vi "Test - Draw Teapot.vi"() -> ()   [LabVIEW 2022 SP3, in "Raster.lvlib"]
uses:
  Raster.lvlib
  3D/Triangle.ctl
  3D/Vertex.ctl
  3D/Vector 3D.ctl
  UV.ctl
  Rectangle Dimensions.ctl
  5ea285c7-be76-47ab-bb95-511c6a9aac96.vi
  d84cddbd-8e40-43c7-a758-6e8d8fd6f2c6.vi
  <vilib>/Utility/High Resolution Relative Seconds.vi
  Sort Points.vi
  Calc P4.vi
  Draw Flat Bottom Filled Triangle.vi
  Draw Flat Top Filled Triangle.vi
  Draw Horizontal Line.vi
  3D/Round Vertex.vi
  Utility/Convert Pixels To Picture.vi/d601d993-a776-4dc8-89c7-357d8398c88c.vi
  Utility/Convert Pixels To Picture.vi/7816d0d6-8e4d-41a2-85ac-ed82f1435763.vi
  Round SGL.vi
  Draw Flat Bottom Filled Triangle.vi/c0c82237-b583-4fc1-b44f-40d02a28ecfd.vi
  Draw Flat Bottom Filled Triangle.vi/53435b12-820c-4aea-aec4-7de16a894549.vi
  Calc Triangle Line Reciprocals.vi
  Global 1.vi
  <vilib>/Utility/colorconv.llb/Color to RGB.vi
  <vilib>/Utility/colorconv.llb/RGB to Color.vi
  <vilib>/picture/picture.llb/Draw Unflattened Pixmap.vi
  <vilib>/picture/picture.llb/Draw True-Color Pixmap.vi
  Utility/Utility.lvlib
  3D/3D.lvlib
panel:
  out "Pixel count":u32
  in  "Teapot":T1[](array[typedef])=[{"Vertex 1"={"Position"={"x"=400.0, "y"=370.36023, "z"=0.9922247}, "UV"={"u"=0.0, "v"=0.0}, "Colour"=12517256}, "Vertex 2"={"Position"={"x"=400.0, "y"=370.5378, "z"=0.99224055}, "UV"={"u"=0.0, "v"=0.0}, "Colour"=12517256}, "Vertex 3"={"Position"={"x"=418.7357, "y"=370.73743, "z"=0.99221843}, "UV"={"u"=0.0, "v"=0.0}, "Colour"=12517256}, "Alpha"=0.0, "Alpha Blending Enabled"=FALSE, "Colour"=11067768}, {"Vertex 1"={"Position"={"x"=400.0, "y"=365.60147, "z"=0.9922195}, "UV"={"u"=0.0, "v"=0.0}, "Colour"=12517256}, "Vertex 2"={"Position"={"x"=400.0, "y"=362.58005, "z"=0.99223673}, "UV"={"u"=0.0, "v"=0.0}, "Colour"=12517256}, "Vertex 3"={"Position"={"x"=381.29703, "y"=362.75687, "z"=0.9922147}, "UV"={"u"=0.0, "v"=0.0}, "Colour"=12517256}, "Alpha"=0.0, "Alpha Blending Enabled"=FALSE, "Colour"=4941110}, {"Vertex 1"={"Position"={"x"=400.0, "y"=370.5378, "z"=0.99224055}, "UV"={"u"=0.0, "v"=0.0}, "Colour"=12517256}, "Vertex 2"={"Position"={"x"=400.0, "y"=370.36023, "z"=0.9922247}, "UV"={"u"=0.0, "v"=0.0}, "Colour"=12517256}, "Vertex 3"={"Position"={"x"=381.39975, "y"=370.55798, "z"=0.99220276}, "UV"={"u"=0.0, "v"=0.0}, "Colour"=12517256}, "Alpha"=0.0, "Alpha Blending Enabled"=FALSE, "Colour"=11067768}, {"Vertex 1"={"Position"={"x"=381.39975, "y"=370.55798, "z"=0.99220276}, "UV"={"u"=0.0, "v"=0.0}, "Colour"=12517256}, "Vertex 2"={"Position"={"x"=381.2643, "y"=370.73743, "z"=0.99221843}, "UV"={"u"=0.0, "v"=0.0}, "Colour"=12517256}, "Vertex 3"={"Position"={"x"=400.0, "y"=370.5378, "z"=0.99224055}, "UV"={"u"=0.0, "v"=0.0}, "Colour"=12517256}, "Alpha"=0.0, "Alpha Blending Enabled"=FALSE, "Colour"=11067768}, {"Vertex 1"={"Position"={"x"=400.0, "y"=362.58005, "z"=0.99223673}, "UV"={"u"=0.0, "v"=0.0}, "Colour"=12517256}, "Vertex 2"={"Position"={"x"=400.0, "y"=365.60147, "z"=0.9922195}, "UV"={"u"=0.0, "v"=0.0}, "Colour"=12517256}, "Vertex 3"={"Position"={"x"=418.5554, "y"=365.78537, "z"=0.9921976}, "UV"={"u"=0.0, "v"=0.0}, "Colour"=12517256}, "Alpha"=0.0, "Alpha Blending Enabled"=FALSE, "Colour"=4941110}, {"Vertex 1"={"Position"={"x"=418.5554, "y"=365.78537, "z"=0.9921976}, "UV"={"u"=0.0, "v"=0.0}, "Colour"=12517256}, "Vertex 2"={"Position"={"x"=418.70297, "y"=362.75687, "z"=0.9922147}, "UV"={"u"=0.0, "v"=0.0}, "Colour"=12517256}, "Vertex 3"={"Position"={"x"=400.0, "y"=362.58005, "z"=0.99223673}, "UV"={"u"=0.0, "v"=0.0}, "Colour"=12517256}, "Alpha"=0.0, "Alpha Blending Enabled"=FALSE, "Colour"=4941110}, {"Vertex 1"={"Position"={"x"=418.7357, "y"=370.73743, "z"=0.99221843}, "UV"={"u"=0.0, "v"=0.0}, "Colour"=12517256}, "Vertex 2"={"Position"={"x"=418.60028, "y"=370.55798, "z"=0.99220276}, "UV"={"u"=0.0, "v"=0.0}, "Colour"=12517256}, "Vertex 3"={"Position"={"x"=400.0, "y"=370.36023, "z"=0.9922247}, "UV"={"u"=0.0, "v"=0.0}, "Colour"=12517256}, "Alpha"=0.0, "Alpha Blending Enabled"=FALSE, "Colour"=11067768}, {"Vertex 1"={"Position"={"x"=400.0, "y"=369.48642, "z"=0.992215}, "UV"={"u"=0.0, "v"=0.0}, "Colour"=12517256}, "Vertex 2"={"Position"={"x"=400.0, "y"=370.36023, "z"=0.9922247}, "UV"={"u"=0.0, "v"=0.0}, "Colour"=12517256}, "Vertex 3"={"Position"={"x"=418.60028, "y"=370.55798, "z"=0.99220276}, "UV"={"u"=0.0, "v"=0.0}, "Colour"=12517256}, "Alpha"=0.0, "Alpha Blending Enabled"=FALSE, "Colour"=12253829}, {"Vertex 1"={"Position"={"x"=400.0, "y"=370.36023, "z"=0.9922247}, "UV"={"u"=0.0, "v"=0.0}, "Colour"=12517256}, "Vertex 2"={"Position"={"x"=400.0, "y"=369.48642, "z"=0.992215}, "UV"={"u"=0.0, "v"=0.0}, "Colour"=12517256}, "Vertex 3"={"Position"={"x"=381.4836, "y"=369.6808, "z"=0.9921931}, "UV"={"u"=0.0, "v"=0.0}, "Colour"=12517256}, "Alpha"=0.0, "Alpha Blending Enabled"=FALSE, "Colour"=12253829}, {"Vertex 1"={"Position"={"x"=381.29703, "y"=362.75687, "z"=0.9922147}, "UV"={"u"=0.0, "v"=0.0}, "Colour"=12517256}, "Vertex 2"={"Position"={"x"=381.4446, "y"=365.78537, "z"=0.9921976}, "UV"={"u"=0.0, "v"=0.0}, "Colour"=12517256}, "Vertex 3"={"Position"={"x"=400.0, "y"=365.60147, "z"=0.9922195}, "UV"={"u"=0.0, "v"=0.0}, "Colour"=12517256}, "Alpha"=0.0, "Alpha Blending Enabled"=FALSE, "Colour"=4941110}, {"Vertex 1"={"Position"={"x"=400.0, "y"=367.90298, "z"=0.9922127}, "UV"={"u"=0.0, "v"=0.0}, "Colour"=12517256}, "Vertex 2"={"Position"={"x"=400.0, "y"=365.60147, "z"=0.9922195}, "UV"={"u"=0.0, "v"=0.0}, "Colour"=12517256}, "Vertex 3"={"Position"={"x"=381.4446, "y"=365.78537, "z"=0.9921976}, "UV"={"u"=0.0, "v"=0.0}, "Colour"=12517256}, "Alpha"=0.0, "Alpha Blending Enabled"=FALSE, "Colour"=6917451}, {"Vertex 1"={"Position"={"x"=400.0, "y"=365.60147, "z"=0.9922195}, "UV"={"u"=0.0, "v"=0.0}, "Colour"=12517256}, "Vertex 2"={"Position"={"x"=400.0, "y"=367.90298, "z"=0.9922127}, "UV"={"u"=0.0, "v"=0.0}, "Colour"=12517256}, "Vertex 3"={"Position"={"x"=418.49722, "y"=368.09274, "z"=0.99219084}, "UV"={"u"=0.0, "v"=0.0}, "Colour"=12517256}, "Alpha"=0.0, "Alpha Blending Enabled"=FALSE, "Colour"=6917451}, {"Vertex 1"={"Position"={"x"=400.0, "y"=367.90298, "z"=0.9922127}, "UV"={"u"=0.0, "v"=0.0}, "Colour"=12517256}, "Vertex 2"={"Position"={"x"=400.0, "y"=369.48642, "z"=0.992215}, "UV"={"u"=0.0, "v"=0.0}, "Colour"=12517256}, "Vertex 3"={"Position"={"x"=418.5164, "y"=369.6808, "z"=0.9921931}, "UV"={"u"=0.0, "v"=0.0}, "Colour"=12517256}, "Alpha"=0.0, "Alpha Blending Enabled"=FALSE, "Colour"=9618536}, {"Vertex 1"={"Position"={"x"=381.4836, "y"=369.6808, "z"=0.9921931}, "UV"={"u"=0.0, "v"=0.0}, "Colour"=12517256}, "Vertex 2"={"Position"={"x"=381.39975, "y"=370.55798, "z"=0.99220276}, "UV"={"u"=0.0, "v"=0.0}, "Colour"=12517256}, "Vertex 3"={"Position"={"x"=400.0, "y"=370.36023, "z"=0.9922247}, "UV"={"u"=0.0, "v"=0.0}, "Colour"=12517256}, "Alpha"=0.0, "Alpha Blending Enabled"=FALSE, "Colour"=12253829}, {"Vertex 1"={"Position"={"x"=400.0, "y"=369.48642, "z"=0.992215}, "UV"={"u"=0.0, "v"=0.0}, "Colour"=12517256}, "Vertex 2"={"Position"={"x"=400.0, "y"=367.90298, "z"=0.9922127}, "UV"={"u"=0.0, "v"=0.0}, "Colour"=12517256}, "Vertex 3"={"Position"={"x"=381.50278, "y"=368.09274, "z"=0.99219084}, "UV"={"u"=0.0, "v"=0.0}, "Colour"=12517256}, "Alpha"=0.0, "Alpha Blending Enabled"=FALSE, "Colour"=9618536}, {"Vertex 1"={"Position"={"x"=418.60028, "y"=370.55798, "z"=0.99220276}, "UV"={"u"=0.0, "v"=0.0}, "Colour"=12517256}, "Vertex 2"={"Position"={"x"=418.5164, "y"=369.6808, "z"=0.9921931}, "UV"={"u"=0.0, "v"=0.0}, "Colour"=12517256}, "Vertex 3"={"Position"={"x"=400.0, "y"=369.48642, "z"=0.992215}, "UV"={"u"=0.0, "v"=0.0}, "Colour"=12517256}, "Alpha"=0.0, "Alpha Blending Enabled"=FALSE, "Colour"=12253829}, {"Vertex 1"={"Position"={"x"=418.49722, "y"=368.09274, "z"=0.99219084}, "UV"={"u"=0.0, "v"=0.0}, "Colour"=12517256}, "Vertex 2"={"Position"={"x"=418.5554, "y"=365.78537, "z"=0.9921976}, "UV"={"u"=0.0, "v"=0.0}, "Colour"=12517256}, "Vertex 3"={"Position"={"x"=400.0, "y"=365.60147, "z"=0.9922195}, "UV"={"u"=0.0, "v"=0.0}, "Colour"=12517256}, "Alpha"=0.0, "Alpha Blending Enabled"=FALSE, "Colour"=6917451}, {"Vertex 1"={"Position"={"x"=381.4446, "y"=365.78537, "z"=0.9921976}, "UV"={"u"=0.0, "v"=0.0}, "Colour"=12517256}, "Vertex 2"={"Position"={"x"=381.50278, "y"=368.09274, "z"=0.99219084}, "UV"={"u"=0.0, "v"=0.0}, "Colour"=12517256}, "Vertex 3"={"Position"={"x"=400.0, "y"=367.90298, "z"=0.9922127}, "UV"={"u"=0.0, "v"=0.0}, "Colour"=12517256}, "Alpha"=0.0, "Alpha Blending Enabled"=FALSE, "Colour"=6917451}, {"Vertex 1"={"Position"={"x"=381.50278, "y"=368.09274, "z"=0.99219084}, "UV"={"u"=0.0, "v"=0.0}, "Colour"=12517256}, "Vertex 2"={"Position"={"x"=381.4836, "y"=369.6808, "z"=0.9921931}, "UV"={"u"=0.0, "v"=0.0}, "Colour"=12517256}, "Vertex 3"={"Position"={"x"=400.0, "y"=369.48642, "z"=0.992215}, "UV"={"u"=0.0, "v"=0.0}, "Colour"=12517256}, "Alpha"=0.0, "Alpha Blending Enabled"=FALSE, "Colour"=9618536}, {"Vertex 1"={"Position"={"x"=418.5164, "y"=369.6808, "z"=0.9921931}, "UV"={"u"=0.0, "v"=0.0}, "Colour"=12517256}, "Vertex 2"={"Position"={"x"=418.49722, "y"=368.09274, "z"=0.99219084}, "UV"={"u"=0.0, "v"=0.0}, "Colour"=12517256}, "Vertex 3"={"Position"={"x"=400.0, "y"=367.90298, "z"=0.9922127}, "UV"={"u"=0.0, "v"=0.0}, "Colour"=12517256}, "Alpha"=0.0, "Alpha Blending Enabled"=FALSE, "Colour"=9618536}, {"Vertex 1"={"Position"={"x"=418.60028, "y"=370.55798, "z"=0.99220276}, "UV"={"u"=0.0, "v"=0.0}, "Colour"=12517256}, "Vertex 2"={"Position"={"x"=418.7357, "y"=370.73743, "z"=0.99221843}, "UV"={"u"=0.0, "v"=0.0}, "Colour"=12517256}, "Vertex 3"={"Position"={"x"=436.73154, "y"=371.323, "z"=0.99215364}, "UV"={"u"=0.0, "v"=0.0}, "Colour"=12517256}, "Alpha"=0.0, "Alpha Blending Enabled"=FALSE, "Colour"=11001975}, {"Vertex 1"={"Position"={"x"=381.4446, "y"=365.78537, "z"=0.9921976}, "UV"={"u"=0.0, "v"=0.0}, "Colour"=12517256}, "Vertex 2"={"Position"={"x"=381.29703, "y"=362.75687, "z"=0.9922147}, "UV"={"u"=0.0, "v"=0.0}, "Colour"=12517256}, "Vertex 3"={"Position"={"x"=363.33307, "y"=363.27545, "z"=0.99214995}, "UV"={"u"=0.0, "v"=0.0}, "Colour"=12517256}, "Alpha"=0.0, "Alpha Blending Enabled"=FALSE, "Colour"=4743475}, {"Vertex 1"={"Position"={"x"=381.2643, "y"=370.73743, "z"=0.99221843}, "UV"={"u"=0.0, "v"=0.0}, "Colour"=12517256}, "Vertex 2"={"Position"={"x"=381.39975, "y"=370.55798, "z"=0.99220276}, "UV"={"u"=0.0, "v"=0.0}, "Colour"=12517256}, "Vertex 3"={"Position"={"x"=363.53616, "y"=371.13776, "z"=0.99213827}, "UV"={"u"=0.0, "v"=0.0}, "Colour"=12517256}, "Alpha"=0.0, "Alpha Blending Enabled"=FALSE, "Colour"=11001975}, {"Vertex 1"={"Position"={"x"=418.70297, "y"=362.75687, "z"=0.9922147}, "UV"={"u"=0.0, "v"=0.0}, "Colour"=12517256}, "Vertex 2"={"Position"={"x"=418.5554, "y"=365.78537, "z"=0.9921976}, "UV"={"u"=0.0, "v"=0.0}, "Colour"=12517256}, "Vertex 3"={"Position"={"x"=436.37515, "y"=366.32462, "z"=0.9921332}, "UV"={"u"=0.0, "v"=0.0}, "Colour"=12517256}, "Alpha"=0.0, "Alpha Blending Enabled"=FALSE, "Colour"=4743475}, {"Vertex 1"={"Position"={"x"=418.5164, "y"=369.6808, "z"=0.9921931}, "UV"={"u"=0.0, "v"=0.0}, "Colour"=12517256}, "Vertex 2"={"Position"={"x"=418.60028, "y"=370.55798, "z"=0.99220276}, "UV"={"u"=0.0, "v"=0.0}, "Colour"=12517256}, "Vertex 3"={"Position"={"x"=436.46384, "y"=371.13776, "z"=0.99213827}, "UV"={"u"=0.0, "v"=0.0}, "Colour"=12517256}, "Alpha"=0.0, "Alpha Blending Enabled"=FALSE, "Colour"=12056195}, {"Vertex 1"={"Position"={"x"=381.39975, "y"=370.55798, "z"=0.99220276}, "UV"={"u"=0.0, "v"=0.0}, "Colour"=12517256}, "Vertex 2"={"Position"={"x"=381.4836, "y"=369.6808, "z"=0.9921931}, "UV"={"u"=0.0, "v"=0.0}, "Colour"=12517256}, "Vertex 3"={"Position"={"x"=363.7018, "y"=370.25076, "z"=0.9921288}, "UV"={"u"=0.0, "v"=0.0}, "Colour"=12517256}, "Alpha"=0.0, "Alpha Blending Enabled"=FALSE, "Colour"=12056195}, {"Vertex 1"={"Position"={"x"=381.50278, "y"=368.09274, "z"=0.99219084}, "UV"={"u"=0.0, "v"=0.0}, "Colour"=12517256}, "Vertex 2"={"Position"={"x"=381.4446, "y"=365.78537, "z"=0.9921976}, "UV"={"u"=0.0, "v"=0.0}, "Colour"=12517256}, "Vertex 3"={"Position"={"x"=363.62485, "y"=366.32462, "z"=0.9921332}, "UV"={"u"=0.0, "v"=0.0}, "Colour"=12517256}, "Alpha"=0.0, "Alpha Blending Enabled"=FALSE, "Colour"=6719817}, {"Vertex 1"={"Position"={"x"=418.5554, "y"=365.78537, "z"=0.9921976}, "UV"={"u"=0.0, "v"=0.0}, "Colour"=12517256}, "Vertex 2"={"Position"={"x"=418.49722, "y"=368.09274, "z"=0.99219084}, "UV"={"u"=0.0, "v"=0.0}, "Colour"=12517256}, "Vertex 3"={"Position"={"x"=436.26022, "y"=368.64917, "z"=0.9921266}, "UV"={"u"=0.0, "v"=0.0}, "Colour"=12517256}, "Alpha"=0.0, "Alpha Blending Enabled"=FALSE, "Colour"=6719817}, {"Vertex 1"={"Position"={"x"=418.49722, "y"=368.09274, "z"=0.99219084}, "UV"={"u"=0.0, "v"=0.0}, "Colour"=12517256}, "Vertex 2"={"Position"={"x"=418.5164, "y"=369.6808, "z"=0.9921931}, "UV"={"u"=0.0, "v"=0.0}, "Colour"=12517256}, "Vertex 3"={"Position"={"x"=436.2982, "y"=370.25076, "z"=0.9921288}, "UV"={"u"=0.0, "v"=0.0}, "Colour"=12517256}, "Alpha"=0.0, "Alpha Blending Enabled"=FALSE, "Colour"=9355110}, {"Vertex 1"={"Position"={"x"=381.4836, "y"=369.6808, "z"=0.9921931}, "UV"={"u"=0.0, "v"=0.0}, "Colour"=12517256}, "Vertex 2"={"Position"={"x"=381.50278, "y"=368.09274, "z"=0.99219084}, "UV"={"u"=0.0, "v"=0.0}, "Colour"=12517256}, "Vertex 3"={"Position"={"x"=363.73975, "y"=368.64917, "z"=0.9921266}, "UV"={"u"=0.0, "v"=0.0}, "Colour"=12517256}, "Alpha"=0.0, "Alpha Blending Enabled"=FALSE, "Colour"=9355110}, {"Vertex 1"={"Position"={"x"=363.53616, "y"=371.13776, "z"=0.99213827}, "UV"={"u"=0.0, "v"=0.0}, "Colour"=12517256}, "Vertex 2"={"Position"={"x"=363.26846, "y"=371.323, "z"=0.99215364}, "UV"={"u"=0.0, "v"=0.0}, "Colour"=12517256}, "Vertex 3"={"Position"={"x"=381.2643, "y"=370.73743, "z"=0.99221843}, "UV"={"u"=0.0, "v"=0.0}, "Colour"=12517256}, "Alpha"=0.0, "Alpha Blending Enabled"=FALSE, "Colour"=11001975}, {"Vertex 1"={"Position"={"x"=436.37515, "y"=366.32462, "z"=0.9921332}, "UV"={"u"=0.0, "v"=0.0}, "Colour"=12517256}, "Vertex 2"={"Position"={"x"=436.66693, "y"=363.27545, "z"=0.99214995}, "UV"={"u"=0.0, "v"=0.0}, "Colour"=12517256}, "Vertex 3"={"Position"={"x"=418.70297, "y"=362.75687, "z"=0.9922147}, "UV"={"u"=0.0, "v"=0.0}, "Colour"=12517256}, "Alpha"=0.0, "Alpha Blending Enabled"=FALSE, "Colour"=4743475}, {"Vertex 1"={"Position"={"x"=436.73154, "y"=371.323, "z"=0.99215364}, "UV"={"u"=0.0, "v"=0.0}, "Colour"=12517256}, "Vertex 2"={"Position"={"x"=436.46384, "y"=371.13776, "z"=0.99213827}, "UV"={"u"=0.0, "v"=0.0}, "Colour"=12517256}, "Vertex 3"={"Position"={"x"=418.60028, "y"=370.55798, "z"=0.99220276}, "UV"={"u"=0.0, "v"=0.0}, "Colour"=12517256}, "Alpha"=0.0, "Alpha Blending Enabled"=FALSE, "Colour"=11001975}, {"Vertex 1"={"Position"={"x"=363.33307, "y"=363.27545, "z"=0.99214995}, "UV"={"u"=0.0, "v"=0.0}, "Colour"=12517256}, "Vertex 2"={"Position"={"x"=363.62485, "y"=366.32462, "z"=0.9921332}, "UV"={"u"=0.0, "v"=0.0}, "Colour"=12517256}, "Vertex 3"={"Position"={"x"=381.4446, "y"=365.78537, "z"=0.9921976}, "UV"={"u"=0.0, "v"=0.0}, "Colour"=12517256}, "Alpha"=0.0, "Alpha Blending Enabled"=FALSE, "Colour"=4743475}, {"Vertex 1"={"Position"={"x"=363.7018, "y"=370.25076, "z"=0.9921288}, "UV"={"u"=0.0, "v"=0.0}, "Colour"=12517256}, "Vertex 2"={"Position"={"x"=363.53616, "y"=371.13776, "z"=0.99213827}, "UV"={"u"=0.0, "v"=0.0}, "Colour"=12517256}, "Vertex 3"={"Position"={"x"=381.39975, "y"=370.55798, "z"=0.99220276}, "UV"={"u"=0.0, "v"=0.0}, "Colour"=12517256}, "Alpha"=0.0, "Alpha Blending Enabled"=FALSE, "Colour"=12056195}, {"Vertex 1"={"Position"={"x"=436.46384, "y"=371.13776, "z"=0.99213827}, "UV"={"u"=0.0, "v"=0.0}, "Colour"=12517256}, "Vertex 2"={"Position"={"x"=436.2982, "y"=370.25076, "z"=0.9921288}, "UV"={"u"=0.0, "v"=0.0}, "Colour"=12517256}, "Vertex 3"={"Position"={"x"=418.5164, "y"=369.6808, "z"=0.9921931}, "UV"={"u"=0.0, "v"=0.0}, "Colour"=12517256}, "Alpha"=0.0, "Alpha Blending Enabled"=FALSE, "Colour"=12056195}, {"Vertex 1"={"Position"={"x"=436.26022, "y"=368.64917, "z"=0.9921266}, "UV"={"u"=0.0, "v"=0.0}, "Colour"=12517256}, "Vertex 2"={"Position"={"x"=436.37515, "y"=366.32462, "z"=0.9921332}, "UV"={"u"=0.0, "v"=0.0}, "Colour"=12517256}, "Vertex 3"={"Position"={"x"=418.5554, "y"=365.78537, "z"=0.9921976}, "UV"={"u"=0.0, "v"=0.0}, "Colour"=12517256}, "Alpha"=0.0, "Alpha Blending Enabled"=FALSE, "Colour"=6719817}, {"Vertex 1"={"Position"={"x"=363.62485, "y"=366.32462, "z"=0.9921332}, "UV"={"u"=0.0, "v"=0.0}, "Colour"=12517256}, "Vertex 2"={"Position"={"x"=363.73975, "y"=368.64917, "z"=0.9921266}, "UV"={"u"=0.0, "v"=0.0}, "Colour"=12517256}, "Vertex 3"={"Position"={"x"=381.50278, "y"=368.09274, "z"=0.99219084}, "UV"={"u"=0.0, "v"=0.0}, "Colour"=12517256}, "Alpha"=0.0, "Alpha Blending Enabled"=FALSE, "Colour"=6719817}, {"Vertex 1"={"Position"={"x"=363.73975, "y"=368.64917, "z"=0.9921266}, "UV"={"u"=0.0, "v"=0.0}, "Colour"=12517256}, "Vertex 2"={"Position"={"x"=363.7018, "y"=370.25076, "z"=0.9921288}, "UV"={"u"=0.0, "v"=0.0}, "Colour"=12517256}, "Vertex 3"={"Position"={"x"=381.4836, "y"=369.6808, "z"=0.9921931}, "UV"={"u"=0.0, "v"=0.0}, "Colour"=12517256}, "Alpha"=0.0, "Alpha Blending Enabled"=FALSE, "Colour"=9355110}, {"Vertex 1"={"Position"={"x"=436.2982, "y"=370.25076, "z"=0.9921288}, "UV"={"u"=0.0, "v"=0.0}, "Colour"=12517256}, "Vertex 2"={"Position"={"x"=436.26022, "y"=368.64917, "z"=0.9921266}, "UV"={"u"=0.0, "v"=0.0}, "Colour"=12517256}, "Vertex 3"={"Position"={"x"=418.49722, "y"=368.09274, "z"=0.99219084}, "UV"={"u"=0.0, "v"=0.0}, "Colour"=12517256}, "Alpha"=0.0, "Alpha Blending Enabled"=FALSE, "Colour"=9355110}, {"Vertex 1"={"Position"={"x"=436.46384, "y"=371.13776, "z"=0.99213827}, "UV"={"u"=0.0, "v"=0.0}, "Colour"=12517256}, "Vertex 2"={"Position"={"x"=436.73154, "y"=371.323, "z"=0.99215364}, "UV"={"u"=0.0, "v"=0.0}, "Colour"=12517256}, "Vertex 3"={"Position"={"x"=454.01846, "y"=372.28268, "z"=0.99204737}, "UV"={"u"=0.0, "v"=0.0}, "Colour"=12517256}, "Alpha"=0.0, "Alpha Blending Enabled"=FALSE, "Colour"=10870134}, {"Vertex 1"={"Position"={"x"=363.62485, "y"=366.32462, "z"=0.9921332}, "UV"={"u"=0.0, "v"=0.0}, "Colour"=12517256}, "Vertex 2"={"Position"={"x"=363.33307, "y"=363.27545, "z"=0.99214995}, "UV"={"u"=0.0, "v"=0.0}, "Colour"=12517256}, "Vertex 3"={"Position"={"x"=346.07788, "y"=364.12534, "z"=0.9920438}, "UV"={"u"=0.0, "v"=0.0}, "Colour"=12517256}, "Alpha"=0.0, "Alpha Blending Enabled"=FALSE, "Colour"=4347951}, {"Vertex 1"={"Position"={"x"=363.26846, "y"=371.323, "z"=0.99215364}, "UV"={"u"=0.0, "v"=0.0}, "Colour"=12517256}, "Vertex 2"={"Position"={"x"=363.53616, "y"=371.13776, "z"=0.99213827}, "UV"={"u"=0.0, "v"=0.0}, "Colour"=12517256}, "Vertex 3"={"Position"={"x"=346.38046, "y"=372.08786, "z"=0.9920326}, "UV"={"u"=0.0, "v"=0.0}, "Colour"=12517256}, "Alpha"=0.0, "Alpha Blending Enabled"=FALSE, "Colour"=10870134}, {"Vertex 1"={"Position"={"x"=436.66693, "y"=363.27545, "z"=0.99214995}, "UV"={"u"=0.0, "v"=0.0}, "Colour"=12517256}, "Vertex 2"={"Position"={"x"=436.37515, "y"=366.32462, "z"=0.9921332}, "UV"={"u"=0.0, "v"=0.0}, "Colour"=12517256}, "Vertex 3"={"Position"={"x"=453.4873, "y"=367.20825, "z"=0.9920277}, "UV"={"u"=0.0, "v"=0.0}, "Colour"=12517256}, "Alpha"=0.0, "Alpha Blending Enabled"=FALSE, "Colour"=4347951}, {"Vertex 1"={"Position"={"x"=436.2982, "y"=370.25076, "z"=0.9921288}, "UV"={"u"=0.0, "v"=0.0}, "Colour"=12517256}, "Vertex 2"={"Position"={"x"=436.46384, "y"=371.13776, "z"=0.99213827}, "UV"={"u"=0.0, "v"=0.0}, "Colour"=12517256}, "Vertex 3"={"Position"={"x"=453.61954, "y"=372.08786, "z"=0.9920326}, "UV"={"u"=0.0, "v"=0.0}, "Colour"=12517256}, "Alpha"=0.0, "Alpha Blending Enabled"=FALSE, "Colour"=11726719}, {"Vertex 1"={"Position"={"x"=363.53616, "y"=371.13776, "z"=0.99213827}, "UV"={"u"=0.0, "v"=0.0}, "Colour"=12517256}, "Vertex 2"={"Position"={"x"=363.7018, "y"=370.25076, "z"=0.9921288}, "UV"={"u"=0.0, "v"=0.0}, "Colour"=12517256}, "Vertex 3"={"Position"={"x"=346.62732, "y"=371.18472, "z"=0.99202347}, "UV"={"u"=0.0, "v"=0.0}, "Colour"=12517256}, "Alpha"=0.0, "Alpha Blending Enabled"=FALSE, "Colour"=11726719}, {"Vertex 1"={"Position"={"x"=363.73975, "y"=368.64917, "z"=0.9921266}, "UV"={"u"=0.0, "v"=0.0}, "Colour"=12517256}, "Vertex 2"={"Position"={"x"=363.62485, "y"=366.32462, "z"=0.9921332}, "UV"={"u"=0.0, "v"=0.0}, "Colour"=12517256}, "Vertex 3"={"Position"={"x"=346.5127, "y"=367.20825, "z"=0.9920277}, "UV"={"u"=0.0, "v"=0.0}, "Colour"=12517256}, "Alpha"=0.0, "Alpha Blending Enabled"=FALSE, "Colour"=6258756}, {"Vertex 1"={"Position"={"x"=436.37515, "y"=366.32462, "z"=0.9921332}, "UV"={"u"=0.0, "v"=0.0}, "Colour"=12517256}, "Vertex 2"={"Position"={"x"=436.26022, "y"=368.64917, "z"=0.9921266}, "UV"={"u"=0.0, "v"=0.0}, "Colour"=12517256}, "Vertex 3"={"Position"={"x"=453.3161, "y"=369.56085, "z"=0.9920214}, "UV"={"u"=0.0, "v"=0.0}, "Colour"=12517256}, "Alpha"=0.0, "Alpha Blending Enabled"=FALSE, "Colour"=6258756}, {"Vertex 1"={"Position"={"x"=436.26022, "y"=368.64917, "z"=0.9921266}, "UV"={"u"=0.0, "v"=0.0}, "Colour"=12517256}, "Vertex 2"={"Position"={"x"=436.2982, "y"=370.25076, "z"=0.9921288}, "UV"={"u"=0.0, "v"=0.0}, "Colour"=12517256}, "Vertex 3"={"Position"={"x"=453.37268, "y"=371.18472, "z"=0.99202347}, "UV"={"u"=0.0, "v"=0.0}, "Colour"=12517256}, "Alpha"=0.0, "Alpha Blending Enabled"=FALSE, "Colour"=8959585}, {"Vertex 1"={"Position"={"x"=363.7018, "y"=370.25076, "z"=0.9921288}, "UV"={"u"=0.0, "v"=0.0}, "Colour"=12517256}, "Vertex 2"={"Position"={"x"=363.73975, "y"=368.64917, "z"=0.9921266}, "UV"={"u"=0.0, "v"=0.0}, "Colour"=12517256}, "Vertex 3"={"Position"={"x"=346.6839, "y"=369.56085, "z"=0.9920214}, "UV"={"u"=0.0, "v"=0.0}, "Colour"=12517256}, "Alpha"=0.0, "Alpha Blending Enabled"=FALSE, "Colour"=8959585}, {"Vertex 1"={"Position"={"x"=346.38046, "y"=372.08786, "z"=0.9920326}, "UV"={"u"=0.0, "v"=0.0}, "Colour"=12517256}, "Vertex 2"={"Position"={"x"=345.98154, "y"=372.28268, "z"=0.99204737}, "UV"={"u"=0.0, "v"=0.0}, "Colour"=12517256}, "Vertex 3"={"Position"={"x"=363.26846, "y"=371.323, "z"=0.99215364}, "UV"={"u"=0.0, "v"=0.0}, "Colour"=12517256}, "Alpha"=0.0, "Alpha Blending Enabled"=FALSE, "Colour"=10870134}, {"Vertex 1"={"Position"={"x"=453.4873, "y"=367.20825, "z"=0.9920277}, "UV"={"u"=0.0, "v"=0.0}, "Colour"=12517256}, "Vertex 2"={"Position"={"x"=453.92212, "y"=364.12534, "z"=0.9920438}, "UV"={"u"=0.0, "v"=0.0}, "Colour"=12517256}, "Vertex 3"={"Position"={"x"=436.66693, "y"=363.27545, "z"=0.99214995}, "UV"={"u"=0.0, "v"=0.0}, "Colour"=12517256}, "Alpha"=0.0, "Alpha Blending Enabled"=FALSE, "Colour"=4347951}, {"Vertex 1"={"Position"={"x"=454.01846, "y"=372.28268, "z"=0.99204737}, "UV"={"u"=0.0, "v"=0.0}, "Colour"=12517256}, "Vertex 2"={"Position"={"x"=453.61954, "y"=372.08786, "z"=0.9920326}, "UV"={"u"=0.0, "v"=0.0}, "Colour"=12517256}, "Vertex 3"={"Position"={"x"=436.46384, "y"=371.13776, "z"=0.99213827}, "UV"={"u"=0.0, "v"=0.0}, "Colour"=12517256}, "Alpha"=0.0, "Alpha Blending Enabled"=FALSE, "Colour"=10870134}, {"Vertex 1"={"Position"={"x"=346.07788, "y"=364.12534, "z"=0.9920438}, "UV"={"u"=0.0, "v"=0.0}, "Colour"=12517256}, "Vertex 2"={"Position"={"x"=346.5127, "y"=367.20825, "z"=0.9920277}, "UV"={"u"=0.0, "v"=0.0}, "Colour"=12517256}, "Vertex 3"={"Position"={"x"=363.62485, "y"=366.32462, "z"=0.9921332}, "UV"={"u"=0.0, "v"=0.0}, "Colour"=12517256}, "Alpha"=0.0, "Alpha Blending Enabled"=FALSE, "Colour"=4347951}, {"Vertex 1"={"Position"={"x"=346.62732, "y"=371.18472, "z"=0.99202347}, "UV"={"u"=0.0, "v"=0.0}, "Colour"=12517256}, "Vertex 2"={"Position"={"x"=346.38046, "y"=372.08786, "z"=0.9920326}, "UV"={"u"=0.0, "v"=0.0}, "Colour"=12517256}, "Vertex 3"={"Position"={"x"=363.53616, "y"=371.13776, "z"=0.99213827}, "UV"={"u"=0.0, "v"=0.0}, "Colour"=12517256}, "Alpha"=0.0, "Alpha Blending Enabled"=FALSE, "Colour"=11726719}, {"Vertex 1"={"Position"={"x"=453.61954, "y"=372.08786, "z"=0.9920326}, "UV"={"u"=0.0, "v"=0.0}, "Colour"=12517256}, "Vertex 2"={"Position"={"x"=453.37268, "y"=371.18472, "z"=0.99202347}, "UV"={"u"=0.0, "v"=0.0}, "Colour"=12517256}, "Vertex 3"={"Position"={"x"=436.2982, "y"=370.25076, "z"=0.9921288}, "UV"={"u"=0.0, "v"=0.0}, "Colour"=12517256}, "Alpha"=0.0, "Alpha Blending Enabled"=FALSE, "Colour"=11726719}, {"Vertex 1"={"Position"={"x"=453.3161, "y"=369.56085, "z"=0.9920214}, "UV"={"u"=0.0, "v"=0.0}, "Colour"=12517256}, "Vertex 2"={"Position"={"x"=453.4873, "y"=367.20825, "z"=0.9920277}, "UV"={"u"=0.0, "v"=0.0}, "Colour"=12517256}, "Vertex 3"={"Position"={"x"=436.37515, "y"=366.32462, "z"=0.9921332}, "UV"={"u"=0.0, "v"=0.0}, "Colour"=12517256}, "Alpha"=0.0, "Alpha Blending Enabled"=FALSE, "Colour"=6258756}, {"Vertex 1"={"Position"={"x"=346.5127, "y"=367.20825, "z"=0.9920277}, "UV"={"u"=0.0, "v"=0.0}, "Colour"=12517256}, "Vertex 2"={"Position"={"x"=346.6839, "y"=369.56085, "z"=0.9920214}, "UV"={"u"=0.0, "v"=0.0}, "Colour"=12517256}, "Vertex 3"={"Position"={"x"=363.73975, "y"=368.64917, "z"=0.9921266}, "UV"={"u"=0.0, "v"=0.0}, "Colour"=12517256}, "Alpha"=0.0, "Alpha Blending Enabled"=FALSE, "Colour"=6258756}, {"Vertex 1"={"Position"={"x"=346.6839, "y"=369.56085, "z"=0.9920214}, "UV"={"u"=0.0, "v"=0.0}, "Colour"=12517256}, "Vertex 2"={"Position"={"x"=346.62732, "y"=371.18472, "z"=0.99202347}, "UV"={"u"=0.0, "v"=0.0}, "Colour"=12517256}, "Vertex 3"={"Position"={"x"=363.7018, "y"=370.25076, "z"=0.9921288}, "UV"={"u"=0.0, "v"=0.0}, "Colour"=12517256}, "Alpha"=0.0, "Alpha Blending Enabled"=FALSE, "Colour"=8959585}, {"Vertex 1"={"Position"={"x"=453.37268, "y"=371.18472, "z"=0.99202347}, "UV"={"u"=0.0, "v"=0.0}, "Colour"=12517256}, "Vertex 2"={"Position"={"x"=453.3161, "y"=369.56085, "z"=0.9920214}, "UV"={"u"=0.0, "v"=0.0}, "Colour"=12517256}, "Vertex 3"={"Position"={"x"=436.26022, "y"=368.64917, "z"=0.9921266}, "UV"={"u"=0.0, "v"=0.0}, "Colour"=12517256}, "Alpha"=0.0, "Alpha Blending Enabled"=FALSE, "Colour"=8959585}, {"Vertex 1"={"Position"={"x"=453.61954, "y"=372.08786, "z"=0.9920326}, "UV"={"u"=0.0, "v"=0.0}, "Colour"=12517256}, "Vertex 2"={"Position"={"x"=454.01846, "y"=372.28268, "z"=0.99204737}, "UV"={"u"=0.0, "v"=0.0}, "Colour"=12517256}, "Vertex 3"={"Position"={"x"=470.57562, "y"=373.61435, "z"=0.99189997}, "UV"={"u"=0.0, "v"=0.0}, "Colour"=12517256}, "Alpha"=0.0, "Alpha Blending Enabled"=FALSE, "Colour"=10672500}, {"Vertex 1"={"Position"={"x"=346.5127, "y"=367.20825, "z"=0.9920277}, "UV"={"u"=0.0, "v"=0.0}, "Colour"=12517256}, "Vertex 2"={"Position"={"x"=346.07788, "y"=364.12534, "z"=0.9920438}, "UV"={"u"=0.0, "v"=0.0}, "Colour"=12517256}, "Vertex 3"={"Position"={"x"=329.55252, "y"=365.30457, "z"=0.99189657}, "UV"={"u"=0.0, "v"=0.0}, "Colour"=12517256}, "Alpha"=0.0, "Alpha Blending Enabled"=FALSE, "Colour"=3755049}, {"Vertex 1"={"Position"={"x"=345.98154, "y"=372.28268, "z"=0.99204737}, "UV"={"u"=0.0, "v"=0.0}, "Colour"=12517256}, "Vertex 2"={"Position"={"x"=346.38046, "y"=372.08786, "z"=0.9920326}, "UV"={"u"=0.0, "v"=0.0}, "Colour"=12517256}, "Vertex 3"={"Position"={"x"=329.95502, "y"=373.40598, "z"=0.991886}, "UV"={"u"=0.0, "v"=0.0}, "Colour"=12517256}, "Alpha"=0.0, "Alpha Blending Enabled"=FALSE, "Colour"=10672500}, {"Vertex 1"={"Position"={"x"=453.92212, "y"=364.12534, "z"=0.9920438}, "UV"={"u"=0.0, "v"=0.0}, "Colour"=12517256}, "Vertex 2"={"Position"={"x"=453.4873, "y"=367.20825, "z"=0.9920277}, "UV"={"u"=0.0, "v"=0.0}, "Colour"=12517256}, "Vertex 3"={"Position"={"x"=469.86905, "y"=368.43405, "z"=0.9918814}, "UV"={"u"=0.0, "v"=0.0}, "Colour"=12517256}, "Alpha"=0.0, "Alpha Blending Enabled"=FALSE, "Colour"=3755049}, {"Vertex 1"={"Position"={"x"=453.37268, "y"=371.18472, "z"=0.99202347}, "UV"={"u"=0.0, "v"=0.0}, "Colour"=12517256}, "Vertex 2"={"Position"={"x"=453.61954, "y"=372.08786, "z"=0.9920326}, "UV"={"u"=0.0, "v"=0.0}, "Colour"=12517256}, "Vertex 3"={"Position"={"x"=470.04498, "y"=373.40598, "z"=0.991886}, "UV"={"u"=0.0, "v"=0.0}, "Colour"=12517256}, "Alpha"=0.0, "Alpha Blending Enabled"=FALSE, "Colour"=11199610}, {"Vertex 1"={"Position"={"x"=346.38046, "y"=372.08786, "z"=0.9920326}, "UV"={"u"=0.0, "v"=0.0}, "Colour"=12517256}, "Vertex 2"={"Position"={"x"=346.62732, "y"=371.18472, "z"=0.99202347}, "UV"={"u"=0.0, "v"=0.0}, "Colour"=12517256}, "Vertex 3"={"Position"={"x"=330.28342, "y"=372.48022, "z"=0.9918774}, "UV"={"u"=0.0, "v"=0.0}, "Colour"=12517256}, "Alpha"=0.0, "Alpha Blending Enabled"=FALSE, "Colour"=11199610}, {"Vertex 1"={"Position"={"x"=346.6839, "y"=369.56085, "z"=0.9920214}, "UV"={"u"=0.0, "v"=0.0}, "Colour"=12517256}, "Vertex 2"={"Position"={"x"=346.5127, "y"=367.20825, "z"=0.9920277}, "UV"={"u"=0.0, "v"=0.0}, "Colour"=12517256}, "Vertex 3"={"Position"={"x"=330.13095, "y"=368.43405, "z"=0.9918814}, "UV"={"u"=0.0, "v"=0.0}, "Colour"=12517256}, "Alpha"=0.0, "Alpha Blending Enabled"=FALSE, "Colour"=5665597}, {"Vertex 1"={"Position"={"x"=453.4873, "y"=367.20825, "z"=0.9920277}, "UV"={"u"=0.0, "v"=0.0}, "Colour"=12517256}, "Vertex 2"={"Position"={"x"=453.3161, "y"=369.56085, "z"=0.9920214}, "UV"={"u"=0.0, "v"=0.0}, "Colour"=12517256}, "Vertex 3"={"Position"={"x"=469.6413, "y"=370.8254, "z"=0.9918754}, "UV"={"u"=0.0, "v"=0.0}, "Colour"=12517256}, "Alpha"=0.0, "Alpha Blending Enabled"=FALSE, "Colour"=5665597}, {"Vertex 1"={"Position"={"x"=453.3161, "y"=369.56085, "z"=0.9920214}, "UV"={"u"=0.0, "v"=0.0}, "Colour"=12517256}, "Vertex 2"={"Position"={"x"=453.37268, "y"=371.18472, "z"=0.99202347}, "UV"={"u"=0.0, "v"=0.0}, "Colour"=12517256}, "Vertex 3"={"Position"={"x"=469.71655, "y"=372.48022, "z"=0.9918774}, "UV"={"u"=0.0, "v"=0.0}, "Colour"=12517256}, "Alpha"=0.0, "Alpha Blending Enabled"=FALSE, "Colour"=8301146}, {"Vertex 1"={"Position"={"x"=346.62732, "y"=371.18472, "z"=0.99202347}, "UV"={"u"=0.0, "v"=0.0}, "Colour"=12517256}, "Vertex 2"={"Position"={"x"=346.6839, "y"=369.56085, "z"=0.9920214}, "UV"={"u"=0.0, "v"=0.0}, "Colour"=12517256}, "Vertex 3"={"Position"={"x"=330.35867, "y"=370.8254, "z"=0.9918754}, "UV"={"u"=0.0, "v"=0.0}, "Colour"=12517256}, "Alpha"=0.0, "Alpha Blending Enabled"=FALSE, "Colour"=8301146}, {"Vertex 1"={"Position"={"x"=329.95502, "y"=373.40598, "z"=0.991886}, "UV"={"u"=0.0, "v"=0.0}, "Colour"=12517256}, "Vertex 2"={"Position"={"x"=329.42438, "y"=373.61435, "z"=0.99189997}, "UV"={"u"=0.0, "v"=0.0}, "Colour"=12517256}, "Vertex 3"={"Position"={"x"=345.98154, "y"=372.28268, "z"=0.99204737}, "UV"={"u"=0.0, "v"=0.0}, "Colour"=12517256}, "Alpha"=0.0, "Alpha Blending Enabled"=FALSE, "Colour"=10672500}, {"Vertex 1"={"Position"={"x"=469.86905, "y"=368.43405, "z"=0.9918814}, "UV"={"u"=0.0, "v"=0.0}, "Colour"=12517256}, "Vertex 2"={"Position"={"x"=470.44748, "y"=365.30457, "z"=0.99189657}, "UV"={"u"=0.0, "v"=0.0}, "Colour"=12517256}, "Vertex 3"={"Position"={"x"=453.92212, "y"=364.12534, "z"=0.9920438}, "UV"={"u"=0.0, "v"=0.0}, "Colour"=12517256}, "Alpha"=0.0, "Alpha Blending Enabled"=FALSE, "Colour"=3755049}, {"Vertex 1"={"Position"={"x"=470.57562, "y"=373.61435, "z"=0.99189997}, "UV"={"u"=0.0, "v"=0.0}, "Colour"=12517256}, "Vertex 2"={"Position"={"x"=470.04498, "y"=373.40598, "z"=0.991886}, "UV"={"u"=0.0, "v"=0.0}, "Colour"=12517256}, "Vertex 3"={"Position"={"x"=453.61954, "y"=372.08786, "z"=0.9920326}, "UV"={"u"=0.0, "v"=0.0}, "Colour"=12517256}, "Alpha"=0.0, "Alpha Blending Enabled"=FALSE, "Colour"=10672500}, {"Vertex 1"={"Position"={"x"=329.55252, "y"=365.30457, "z"=0.99189657}, "UV"={"u"=0.0, "v"=0.0}, "Colour"=12517256}, "Vertex 2"={"Position"={"x"=330.13095, "y"=368.43405, "z"=0.9918814}, "UV"={"u"=0.0, "v"=0.0}, "Colour"=12517256}, "Vertex 3"={"Position"={"x"=346.5127, "y"=367.20825, "z"=0.9920277}, "UV"={"u"=0.0, "v"=0.0}, "Colour"=12517256}, "Alpha"=0.0, "Alpha Blending Enabled"=FALSE, "Colour"=3755049}, {"Vertex 1"={"Position"={"x"=330.28342, "y"=372.48022, "z"=0.9918774}, "UV"={"u"=0.0, "v"=0.0}, "Colour"=12517256}, "Vertex 2"={"Position"={"x"=329.95502, "y"=373.40598, "z"=0.991886}, "UV"={"u"=0.0, "v"=0.0}, "Colour"=12517256}, "Vertex 3"={"Position"={"x"=346.38046, "y"=372.08786, "z"=0.9920326}, "UV"={"u"=0.0, "v"=0.0}, "Colour"=12517256}, "Alpha"=0.0, "Alpha Blending Enabled"=FALSE, "Colour"=11199610}, {"Vertex 1"={"Position"={"x"=470.04498, "y"=373.40598, "z"=0.991886}, "UV"={"u"=0.0, "v"=0.0}, "Colour"=12517256}, "Vertex 2"={"Position"={"x"=469.71655, "y"=372.48022, "z"=0.9918774}, "UV"={"u"=0.0, "v"=0.0}, "Colour"=12517256}, "Vertex 3"={"Position"={"x"=453.37268, "y"=371.18472, "z"=0.99202347}, "UV"={"u"=0.0, "v"=0.0}, "Colour"=12517256}, "Alpha"=0.0, "Alpha Blending Enabled"=FALSE, "Colour"=11199610}, {"Vertex 1"={"Position"={"x"=469.6413, "y"=370.8254, "z"=0.9918754}, "UV"={"u"=0.0, "v"=0.0}, "Colour"=12517256}, "Vertex 2"={"Position"={"x"=469.86905, "y"=368.43405, "z"=0.9918814}, "UV"={"u"=0.0, "v"=0.0}, "Colour"=12517256}, "Vertex 3"={"Position"={"x"=453.4873, "y"=367.20825, "z"=0.9920277}, "UV"={"u"=0.0, "v"=0.0}, "Colour"=12517256}, "Alpha"=0.0, "Alpha Blending Enabled"=FALSE, "Colour"=5665597}, {"Vertex 1"={"Position"={"x"=330.13095, "y"=368.43405, "z"=0.9918814}, "UV"={"u"=0.0, "v"=0.0}, "Colour"=12517256}, "Vertex 2"={"Position"={"x"=330.35867, "y"=370.8254, "z"=0.9918754}, "UV"={"u"=0.0, "v"=0.0}, "Colour"=12517256}, "Vertex 3"={"Position"={"x"=346.6839, "y"=369.56085, "z"=0.9920214}, "UV"={"u"=0.0, "v"=0.0}, "Colour"=12517256}, "Alpha"=0.0, "Alpha Blending Enabled"=FALSE, "Colour"=5665597}, {"Vertex 1"={"Position"={"x"=330.35867, "y"=370.8254, "z"=0.9918754}, "UV"={"u"=0.0, "v"=0.0}, "Colour"=12517256}, "Vertex 2"={"Position"={"x"=330.28342, "y"=372.48022, "z"=0.9918774}, "UV"={"u"=0.0, "v"=0.0}, "Colour"=12517256}, "Vertex 3"={"Position"={"x"=346.62732, "y"=371.18472, "z"=0.99202347}, "UV"={"u"=0.0, "v"=0.0}, "Colour"=12517256}, "Alpha"=0.0, "Alpha Blending Enabled"=FALSE, "Colour"=8301146}, {"Vertex 1"={"Position"={"x"=469.71655, "y"=372.48022, "z"=0.9918774}, "UV"={"u"=0.0, "v"=0.0}, "Colour"=12517256}, "Vertex 2"={"Position"={"x"=469.6413, "y"=370.8254, "z"=0.9918754}, "UV"={"u"=0.0, "v"=0.0}, "Colour"=12517256}, "Vertex 3"={"Position"={"x"=453.3161, "y"=369.56085, "z"=0.9920214}, "UV"={"u"=0.0, "v"=0.0}, "Colour"=12517256}, "Alpha"=0.0, "Alpha Blending Enabled"=FALSE, "Colour"=8301146}, {"Vertex 1"={"Position"={"x"=470.04498, "y"=373.40598, "z"=0.991886}, "UV"={"u"=0.0, "v"=0.0}, "Colour"=12517256}, "Vertex 2"={"Position"={"x"=470.57562, "y"=373.61435, "z"=0.99189997}, "UV"={"u"=0.0, "v"=0.0}, "Colour"=12517256}, "Vertex 3"={"Position"={"x"=486.3295, "y"=375.32452, "z"=0.9917106}, "UV"={"u"=0.0, "v"=0.0}, "Colour"=12517256}, "Alpha"=0.0, "Alpha Blending Enabled"=FALSE, "Colour"=10409073}, {"Vertex 1"={"Position"={"x"=330.13095, "y"=368.43405, "z"=0.9918814}, "UV"={"u"=0.0, "v"=0.0}, "Colour"=12517256}, "Vertex 2"={"Position"={"x"=329.55252, "y"=365.30457, "z"=0.99189657}, "UV"={"u"=0.0, "v"=0.0}, "Colour"=12517256}, "Vertex 3"={"Position"={"x"=313.8309, "y"=366.81888, "z"=0.9917075}, "UV"={"u"=0.0, "v"=0.0}, "Colour"=12517256}, "Alpha"=0.0, "Alpha Blending Enabled"=FALSE, "Colour"=2964768}, {"Vertex 1"={"Position"={"x"=329.42438, "y"=373.61435, "z"=0.99189997}, "UV"={"u"=0.0, "v"=0.0}, "Colour"=12517256}, "Vertex 2"={"Position"={"x"=329.95502, "y"=373.40598, "z"=0.991886}, "UV"={"u"=0.0, "v"=0.0}, "Colour"=12517256}, "Vertex 
